vi "Digitally_VI.vi"() -> ()   [LabVIEW 2019]
panel:
  out "Numeric 2":dbl
  in  "Numeric":dbl
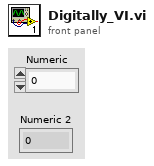
[diagram p1: front panel]
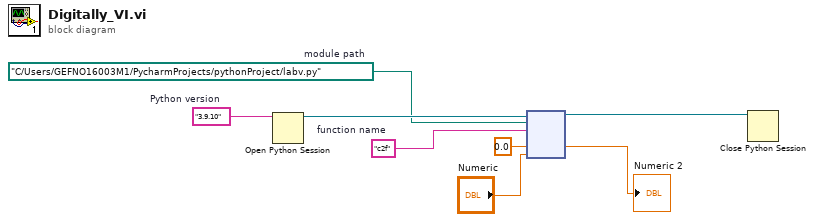
[diagram p0: block diagram]
diagram:
  w5 = "c2f"  # function name
  w6 = path "C:/Users/GEFNO16003M1/PycharmProjects/pythonProject/labv.py"  # module path
  w8 = "3.9.10"  # Python version
  n1 = Open Python Session(python version=w8) -> (session out=w7:refnum<k35>)  [unwired: 2 in, 1 out]
  n2 = node ("Python Node")(w7, w6, w5, 0.0, "Numeric") -> (w3:refnum<k35>, →"Numeric 2":dbl)  [unwired: 2 in, 3 out]
  n3 = Close Python Session(session in=w3) -> ()  [unwired: 1 in, 1 out]
